vi "Clear.vi"(8 "error in (no error)":errorcluster, 11 "XML Report in":refnum<class "Report.lvclass">) -> (0 "error out":errorcluster)   [LabVIEW 2020, in "Report Generation.lvlib" / "Report.lvclass"]
uses:
  Report.lvclass
  Report.lvclass/Report.ctl
  Report Generator/Report Generator.lvclass
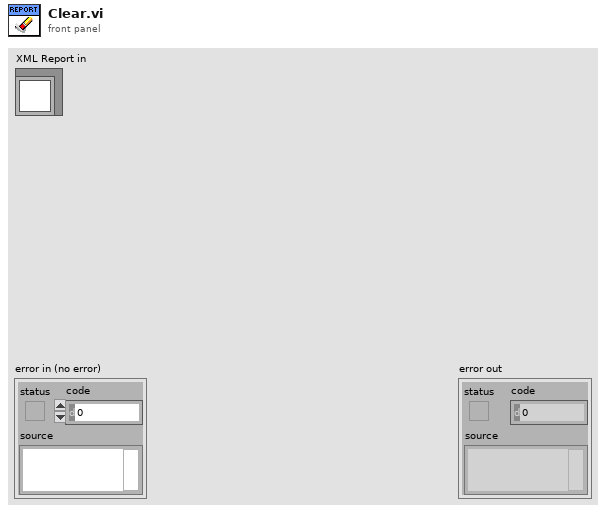
[diagram p1: front panel]
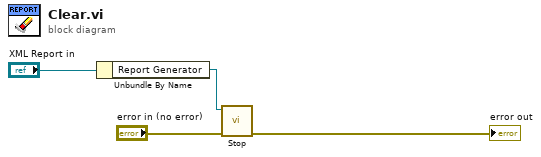
[diagram p0: block diagram]
diagram:
  n1 = Unbundle By Name("XML Report in") -> ("Report Generator"=w3:refnum<class "Report Generator.lvclass">)
  n2 = call "Stop.vi"("error in (no error)"="error in (no error)", "Report Generator In"=w3) -> ("error out"=→"error out":errorcluster)  [unwired: 8 in, 1 out]
